vi "GU List Menu Selection.vi"(8 "error in":errorcluster, 10 "ItemTag":string, 11 "CtlRef":refnum<vi>) -> (0 "error out":errorcluster, 2 "Selected GU":i32[](array[numeric]))   [LabVIEW 2020, in "GUCalibration2.lvlib"]
uses:
  GUCalibration2.lvlib
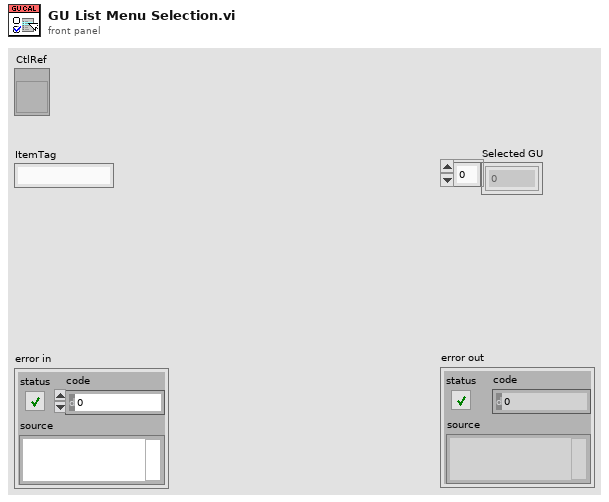
[diagram p1: front panel]
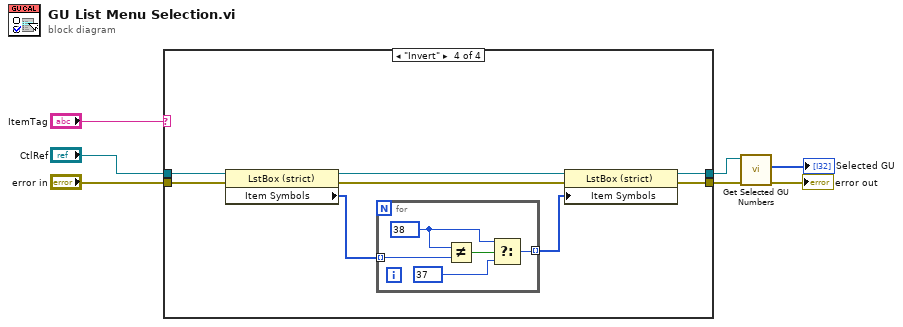
[diagram p0: block diagram]
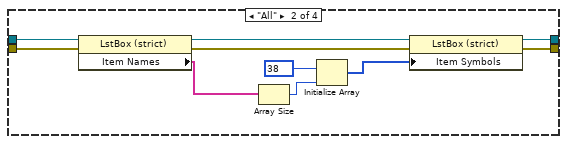
[diagram p3: hidden frame]
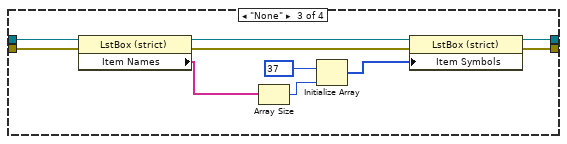
[diagram p4: hidden frame]
diagram:
  n1 = case shown="\"Invert\"" "ItemTag" {
    tunnel: "error in" -> [w9 w18 w27 w34]
    tunnel: "CtlRef" -> [w8 w19 w28 w35]
    tunnel: [w9 w11 w20 w31] -> w4
    tunnel: [w8 w10 w28 w35] -> w3
    frame "False", Default {
    }
    frame "All" {
      n2 = property class="LstBox (strict)"(reference=w19, error in=w18) -> (reference out=w13:refnum<vi>, error out=w14:errorcluster, "Item Names"=w17:string[])
      n3 = Array Size(array=w17) -> (size(s)=w16:i32)
      n4 = Initialize Array(38, w16) -> (w12:i32[])
      n5 = property class="LstBox (strict)"(reference=w13, error in=w14, "Item Symbols"=w12) -> (reference out=w10:refnum<vi>, error out=w11:errorcluster)
    }
    frame "None" {
      n6 = property class="LstBox (strict)"(reference=w28, error in=w27) -> (reference out=w22:refnum<vi>, error out=w23:errorcluster, "Item Names"=w26:string[])
      n7 = Array Size(array=w26) -> (size(s)=w25:i32)
      n8 = Initialize Array(37, w25) -> (w21:i32[])
      n9 = property class="LstBox (strict)"(reference=w22, error in=w23, "Item Symbols"=w21) -> (error out=w20:errorcluster)  [unwired: 1 out]
    }
    frame "Invert" {
      n10 = property class="LstBox (strict)"(reference=w35, error in=w34) -> (reference out=w32:refnum<vi>, error out=w33:errorcluster, "Item Symbols"=w30:i32[])
      n11 = for {
        tunnel: w30 -> [w40] mode=indexing
        tunnel: [w37] -> w29 mode=indexing
        w38 = 38
        n12 = Not Equal?(x=w38, y=w40) -> (x != y?=w39:bool)
        n13 = Select(t=w38, s=w39, f=37) -> (s? t:f=w37:i32)
      }
      n14 = property class="LstBox (strict)"(reference=w32, error in=w33, "Item Symbols"=w29) -> (error out=w31:errorcluster)  [unwired: 1 out]
    }
  }
  n15 = call "Get Selected GU Numbers.vi"("error in"=w4, "Listbox Refnum"=w3) -> ("error out"=→"error out":errorcluster, "Selected GU"=→"Selected GU":i32[])  [unwired: 8 in]
